vi "Read All Pulse.vi"(8 "error in":errorcluster, 11 "Electronic Load in":refnum<class "Electronic Load.lvclass">) -> (0 "error out":errorcluster, 2 "Trigger Settings All":T1, 3 "Electronic Load out":refnum<class "Electronic Load.lvclass">)   [LabVIEW 2019, in "Electronic Load.lvlib" / "Electronic Load.lvclass"]
uses:
  Library/Electronic Load.lvclass
  Custom Controls/Trigger Settings.ctl
  Custom Controls/E-Load Mode.ctl
  Library/Electronic Load.lvclass/Electronic Load.ctl
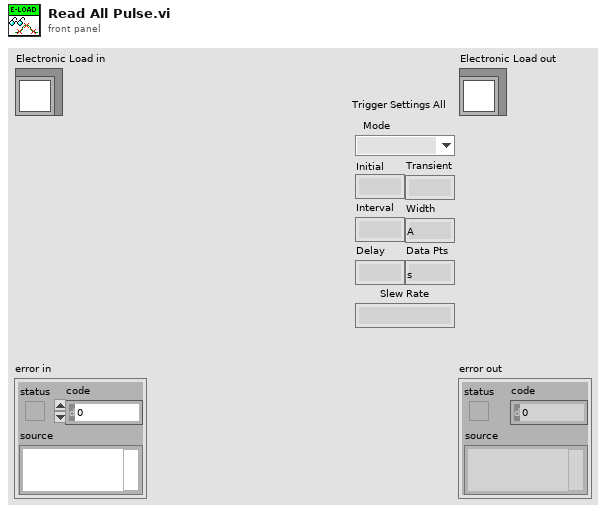
[diagram p1: front panel]
types:
  T1 = typedef "Electronic Load.lvlib/Electronic Load.lvclass/Trigger Settings.ctl" = cluster{"Mode":T2, "Initial":dbl, "Transient":dbl, "Interval":dbl, "Width":dbl, "Delay":dbl, "Data Pts":i32, "Slew Rate":dbl}
  T2 = typedef "Electronic Load.lvlib/Electronic Load.lvclass/E-Load Mode.ctl" = enum16{"Current", "Resistance", "Voltage"}
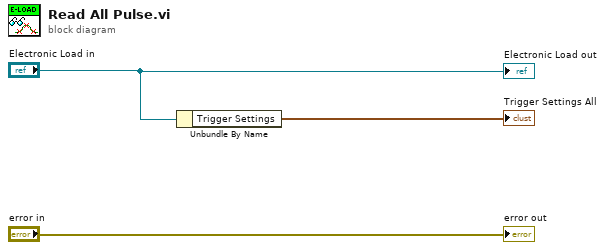
[diagram p0: block diagram]
diagram:
  n1 = Unbundle By Name("Electronic Load in") -> ("Trigger Settings"=→"Trigger Settings All":T1)
  "error out" <- "error in"
  "Electronic Load out" <- "Electronic Load in"
